vi "Left or right.vi"() -> (2 "New target position (units)":dbl, 3 "String":string)   [LabVIEW 2013]
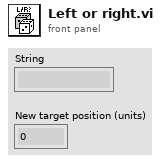
[diagram p1: front panel]
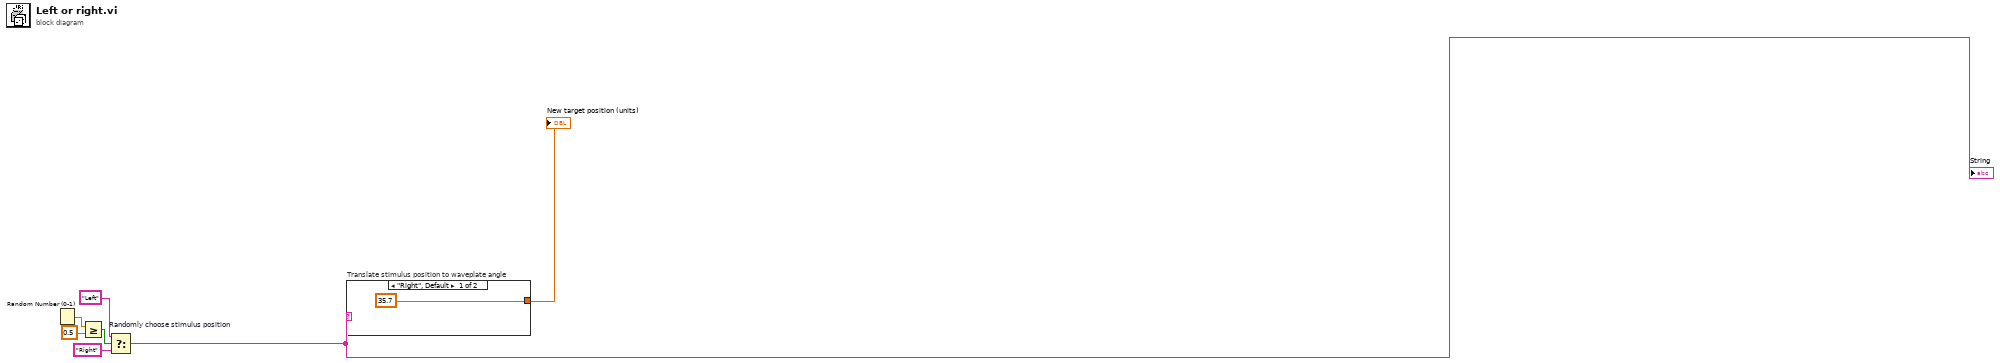
[diagram p0: block diagram]
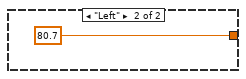
[diagram p2: hidden frame]
diagram:
  n1 = Random Number (0-1)() -> (number: 0 to 1=w5:dbl)
  n2 = Greater Or Equal?(x=w5, y=0.5) -> (x >= y?=w3:bool)
  n3 = Select "Randomly choose stimulus position"(t="Left", s=w3, f="Right") -> (s? t:f=w6:string)
  "String" <- w6
  n4 = case "Translate stimulus position to waveplate angle" shown="\"Right\", Default" w6 {
    tunnel: [35.7 ("New target position (units)") 80.7 ("New target position (units)")] -> w7
    frame "Right", Default {
    }
    frame "Left" {
    }
  }
  "New target position (units)" <- w7
